vi "LDA_U16_data_header.vi"() -> (0 "Output string":string)   [LabVIEW 2015]
uses:
  Globals/Meas_global.vi
  Globals/LDA_meas_global_1.vi
  Globals/LDA_meas_global_2.vi
panel:
  out "length":i32
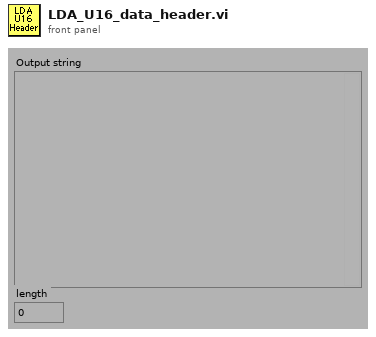
[diagram p1: front panel]
types:
  T1 = typedef "LDA_Setup.ctl" = cluster{"dimensions":enum16{"1D", "2D"}, "Analogue Freq Multiplier":dbl}
  T2 = typedef "BSA_Type.ctl" = enum16{"57N11", "BSA F60"}
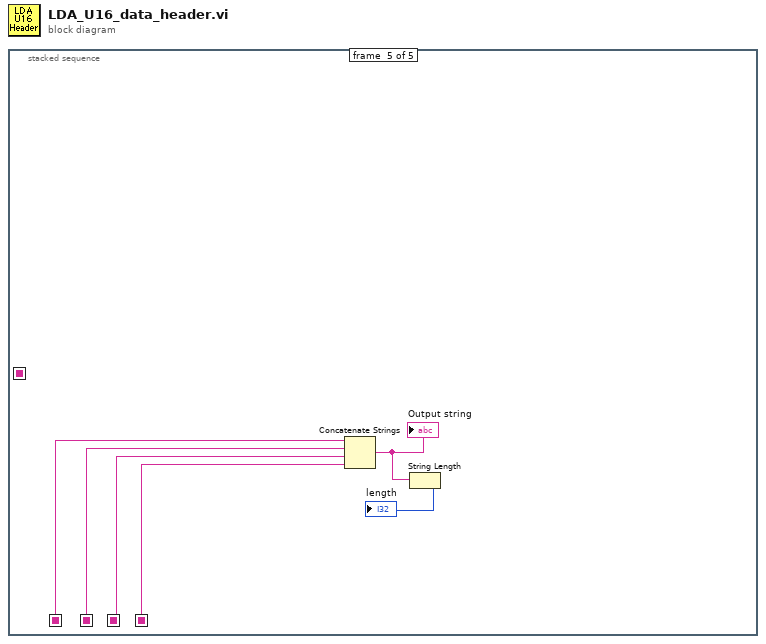
[diagram p0: block diagram]
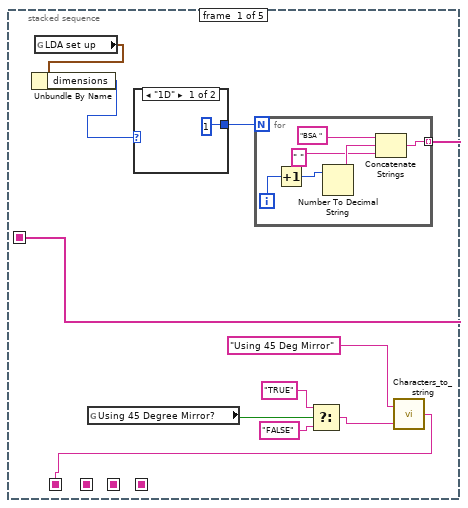
[diagram p2: hidden frame]
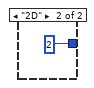
[diagram p3: hidden frame]
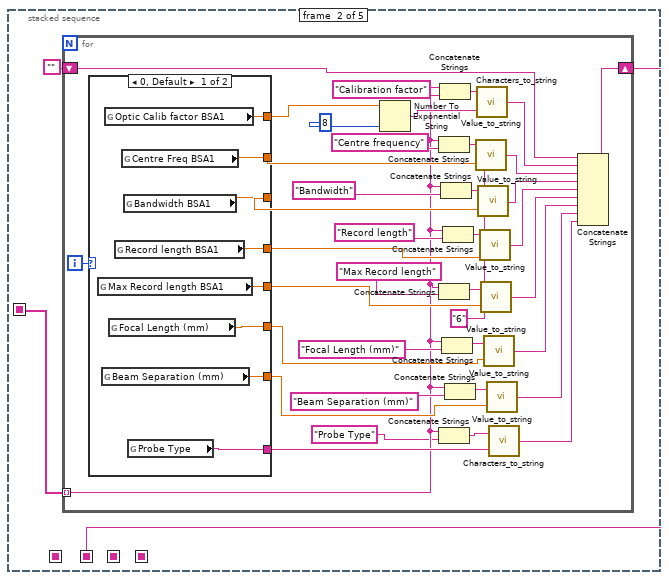
[diagram p4: hidden frame]
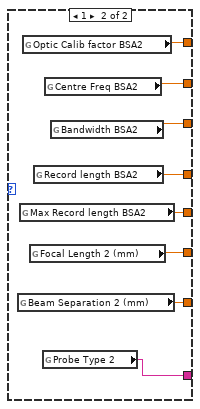
[diagram p5: hidden frame]
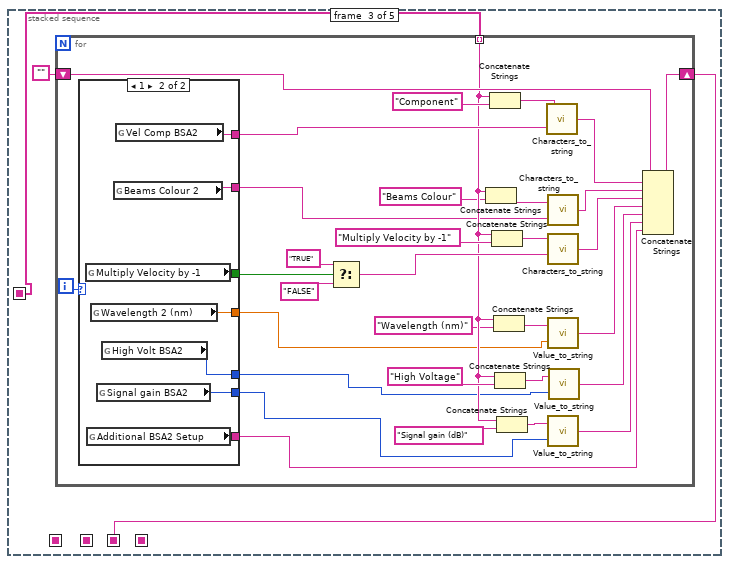
[diagram p6: hidden frame]
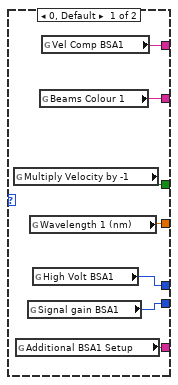
[diagram p7: hidden frame]
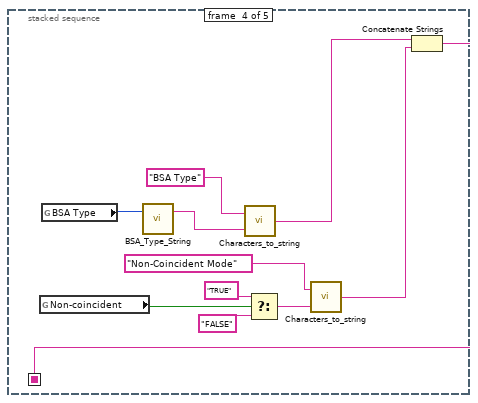
[diagram p8: hidden frame]
diagram:
  n1 = stacked-sequence {
    seq-local: [_ w20 _ _ _] -> [_ _ _ _ w142]
    seq-local: [_ _ w78 _ _] -> [_ _ _ _ w141]
    seq-local: [w10 _ _ _ _] -> [_ w19 w77 _ _]
    seq-local: [_ _ _ w136 _] -> [_ _ _ _ w138]
    seq-local: [w1 _ _ _ _] -> [_ _ _ _ w137]
    frame #0 {
      n2 = global read "Meas_global.vi" "LDA set up"() -> (w8:T1)
      n3 = Unbundle By Name(w8) -> ("dimensions"=w7:enum16{"1D", "2D"})
      n4 = global read "LDA_meas_global_1.vi" "Using 45 Degree Mirror?"() -> (w3:bool)
      n5 = case shown="\"1D\"" w7 {
        tunnel: [1 2] -> w9
        frame "1D" {
        }
        frame "2D" {
        }
      }
      n6 = for {
        N: w9 -> [_]
        tunnel: [w15] -> w10 mode=indexing
        i -> [w13]
        n7 = Increment(x=w13) -> (x+1=w16:i32)
        n8 = Number To Decimal String(number=w16) -> (decimal integer string=w18:string)  [unwired: 1 out]
        n9 = Concatenate Strings("BSA ", w18, " ") -> (w15:string)
      }
      n10 = Select(t="TRUE", s=w3, f="FALSE") -> (s? t:f=w4:string)
      n11 = call "Characters_to_string.vi"("Characters to write"=w4, "Label for characters"="Using 45 Deg Mirror") -> ("Output string"=w1:string)
    }
    frame #1 {
      n12 = for {
        shift-right: [w58] -> w20
        shift-left: "" -> [w59]
        tunnel: w19 -> [w24] mode=indexing
        i -> [w60]
        w38 = "6" ("precision")
        n13 = case shown="0, Default" w60 {
          tunnel: [w68 w73] -> w36
          tunnel: [w67 w74] -> w51
          tunnel: [w66 w75] -> w52
          tunnel: [w65 w76] -> w53
          tunnel: [w64 w72] -> w40
          tunnel: [w63 w70] -> w29
          tunnel: [w62 w71] -> w28
          tunnel: [w61 w69] -> w26
          frame 0, Default {
            n14 = global read "LDA_meas_global_1.vi" "Max Record length BSA1"() -> (w64:dbl)
            n15 = global read "LDA_meas_global_1.vi" "Beam Separation (mm)"() -> (w62:dbl)
            n16 = global read "LDA_meas_global_1.vi" "Optic Calib factor BSA1"() -> (w68:dbl)
            n17 = global read "LDA_meas_global_1.vi" "Focal Length (mm)"() -> (w63:dbl)
            n18 = global read "LDA_meas_global_1.vi" "Record length BSA1"() -> (w65:dbl)
            n19 = global read "LDA_meas_global_1.vi" "Centre Freq BSA1"() -> (w67:dbl)
            n20 = global read "LDA_meas_global_1.vi" "Bandwidth BSA1"() -> (w66:dbl)
            n21 = global read "LDA_meas_global_1.vi" "Probe Type"() -> (w61:string)
          }
          frame 1 {
            n22 = global read "LDA_meas_global_2.vi" "Beam Separation 2 (mm)"() -> (w71:dbl)
            n23 = global read "LDA_meas_global_2.vi" "Max Record length BSA2"() -> (w72:dbl)
            n24 = global read "LDA_meas_global_2.vi" "Optic Calib factor BSA2"() -> (w73:dbl)
            n25 = global read "LDA_meas_global_2.vi" "Focal Length 2 (mm)"() -> (w70:dbl)
            n26 = global read "LDA_meas_global_2.vi" "Record length BSA2"() -> (w76:dbl)
            n27 = global read "LDA_meas_global_2.vi" "Probe Type 2"() -> (w69:string)
            n28 = global read "LDA_meas_global_2.vi" "Centre Freq BSA2"() -> (w74:dbl)
            n29 = global read "LDA_meas_global_2.vi" "Bandwidth BSA2"() -> (w75:dbl)
          }
        }
        n30 = Number To Exponential String(number=w36, precision (6)=i16 8) -> (E-format string=w35:string)  [unwired: 2 out]
        n31 = Concatenate Strings(w24, "Centre frequency") -> (w56:string)
        n32 = Concatenate Strings(w24, "Max Record length") -> (w41:string)
        n33 = Concatenate Strings(w24, "Probe Type" ("Label for characters")) -> (w25:string)
        n34 = Concatenate Strings(w24, "Calibration factor") -> (w57:string)
        n35 = Concatenate Strings(w24, "Bandwidth") -> (w55:string)
        n36 = Concatenate Strings(w24, "Focal Length (mm)" ("Label for characters")) -> (w34:string)
        n37 = Concatenate Strings(w24, "Record length") -> (w54:string)
        n38 = Concatenate Strings(w24, "Beam Separation (mm)" ("Label for characters")) -> (w33:string)
        n39 = call "Value_to_string.vi"("precision"=w38, "Value"=w51, "Label for value"=w56) -> ("Output string"=w49:string)
        n40 = call "Characters_to_string.vi"("Characters to write"=w35, "Label for characters"=w57) -> ("Output string"=w50:string)
        n41 = call "Value_to_string.vi"("precision"=w38, "Value"=w52, "Label for value"=w55) -> ("Output string"=w48:string)
        n42 = call "Value_to_string.vi"("precision"=w38, "Value"=w53, "Label for value"=w54) -> ("Output string"=w43:string)
        n43 = call "Value_to_string.vi"("precision"=w38, "Value"=w40, "Label for value"=w41) -> ("Output string"=w39:string)
        n44 = call "Value_to_string.vi"("Value"=w29, "Label for value"=w34) -> ("Output string"=w30:string)  [unwired: 1 in]
        n45 = call "Value_to_string.vi"("Value"=w28, "Label for value"=w33) -> ("Output string"=w27:string)  [unwired: 1 in]
        n46 = call "Characters_to_string.vi"("Characters to write"=w26, "Label for characters"=w25) -> ("Output string"=w22:string)
        n47 = Concatenate Strings(w59, w50, w49, w48, w43, w39, w30, w27, w22) -> (w58:string)
      }
    }
    frame #2 {
      n48 = for {
        shift-right: [w109] -> w78
        shift-left: "" -> [w110]
        tunnel: w77 -> [w90] mode=indexing
        i -> [w111]
        n49 = case shown="1" w111 {
          tunnel: [w118 w125] -> w80
          tunnel: [w117 w124] -> w105
          tunnel: [w116 w123] -> w102
          tunnel: [w114 w122] -> w84
          tunnel: [w115 w121] -> w83
          tunnel: [w113 w120] -> w82
          tunnel: [w112 w119] -> w81
          frame 0, Default {
            n50 = global read "LDA_meas_global_1.vi" "Multiply Velocity by -1"() -> (w116:bool)
            n51 = global read "LDA_meas_global_1.vi" "Additional BSA1 Setup"() -> (w113:string)
            n52 = global read "LDA_meas_global_1.vi" "Signal gain BSA1"() -> (w114:i16)
            n53 = global read "LDA_meas_global_1.vi" "Wavelength 1 (nm)"() -> (w112:dbl)
            n54 = global read "LDA_meas_global_1.vi" "High Volt BSA1"() -> (w115:i16)
            n55 = global read "LDA_meas_global_1.vi" "Beams Colour 1"() -> (w118:string)
            n56 = global read "LDA_meas_global_1.vi" "Vel Comp BSA1"() -> (w117:string)
          }
          frame 1 {
            n57 = global read "LDA_meas_global_2.vi" "Multiply Velocity by -1"() -> (w123:bool)
            n58 = global read "LDA_meas_global_2.vi" "Additional BSA2 Setup"() -> (w120:string)
            n59 = global read "LDA_meas_global_2.vi" "Wavelength 2 (nm)"() -> (w119:dbl)
            n60 = global read "LDA_meas_global_2.vi" "Signal gain BSA2"() -> (w122:i16)
            n61 = global read "LDA_meas_global_2.vi" "High Volt BSA2"() -> (w121:i16)
            n62 = global read "LDA_meas_global_2.vi" "Beams Colour 2"() -> (w125:string)
            n63 = global read "LDA_meas_global_2.vi" "Vel Comp BSA2"() -> (w124:string)
          }
        }
        n64 = Select(t="TRUE" ("y"), s=w102, f="FALSE" ("y")) -> (s? t:f=w99:string)
        n65 = Concatenate Strings(w90, "Beams Colour" ("string")) -> (w96:string)
        n66 = Concatenate Strings(w90, "Component") -> (w108:string)
        n67 = Concatenate Strings(w90, "Multiply Velocity by -1") -> (w103:string)
        n68 = Concatenate Strings(w90, "Wavelength (nm)") -> (w95:string)
        n69 = Concatenate Strings(w90, "High Voltage") -> (w94:string)
        n70 = Concatenate Strings(w90, "Signal gain (dB)") -> (w93:string)
        n71 = call "Characters_to_string.vi"("Characters to write"=w105, "Label for characters"=w108) -> ("Output string"=w107:string)
        n72 = call "Characters_to_string.vi"("Characters to write"=w80, "Label for characters"=w96) -> ("Output string"=w97:string)
        n73 = call "Characters_to_string.vi"("Characters to write"=w99, "Label for characters"=w103) -> ("Output string"=w98:string)
        n74 = call "Value_to_string.vi"("Value"=w81, "Label for value"=w95) -> ("Output string"=w87:string)  [unwired: 1 in]
        n75 = call "Value_to_string.vi"("Value"=w84, "Label for value"=w93) -> ("Output string"=w89:string)  [unwired: 1 in]
        n76 = call "Value_to_string.vi"("Value"=w83, "Label for value"=w94) -> ("Output string"=w88:string)  [unwired: 1 in]
        n77 = Concatenate Strings(w110, w107, w97, w98, w87, w88, w89, w82) -> (w109:string)
      }
    }
    frame #3 {
      n78 = global read "LDA_meas_global_1.vi" "Non-coincident"() -> (w129:bool)
      n79 = global read "LDA_meas_global_1.vi" "BSA Type"() -> (w135:T2)
      n80 = call "BSA_Type_String.vi"("BSA Type"=w135) -> ("BSA String Out"=w134:string)  [unwired: 1 in, 1 out]
      n81 = call "Characters_to_string.vi"("Characters to write"=w134, "Label for characters"="BSA Type") -> ("Output string"=w133:string)
      n82 = Select(t="TRUE" ("y"), s=w129, f="FALSE" ("y")) -> (s? t:f=w128:string)
      n83 = call "Characters_to_string.vi"("Characters to write"=w128, "Label for characters"="Non-Coincident Mode") -> ("Output string"=w127:string)
      n84 = Concatenate Strings(w133, w127) -> (w136:string)
    }
    frame #4 {
      n85 = Concatenate Strings(w137, w142, w141, w138) -> (w139:string)
      "Output string" <- w139
      n86 = String Length(string=w139) -> (length=→"length":i32)
    }
  }
